vi "Create.vi"(8 "error in (no error)":errorcluster, 10 "Number of Executors":i32) -> (0 "error out":errorcluster, 3 "Executor":refnum<class "Executor.lvclass">)   [LabVIEW 2014, in "Executor.lvclass"]
uses:
  Executor.lvclass
  Controls/Executor Status - STYP.ctl
  Controls/Executor Data - STYP.ctl
  Controls/Job Results - STYP.ctl
  <vilib>/ActorFramework/Message Enqueuer/Message Enqueuer.lvclass
  Executor.lvclass/Executor.ctl
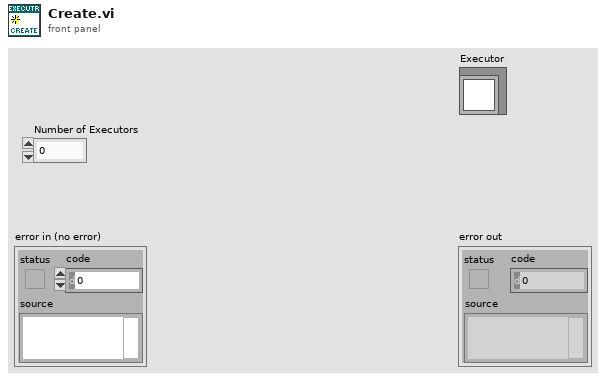
[diagram p1: front panel]
types:
  T1 = typedef "Executor Data - STYP.ctl" = cluster{"Status":T2, "Result Queue":refnum<queue>, "Actor Enquerer":refnum<class "Message Enqueuer.lvclass">}
  T2 = typedef "Executor Status - STYP.ctl" = cluster{"Executor Name":string, "Status":bool}
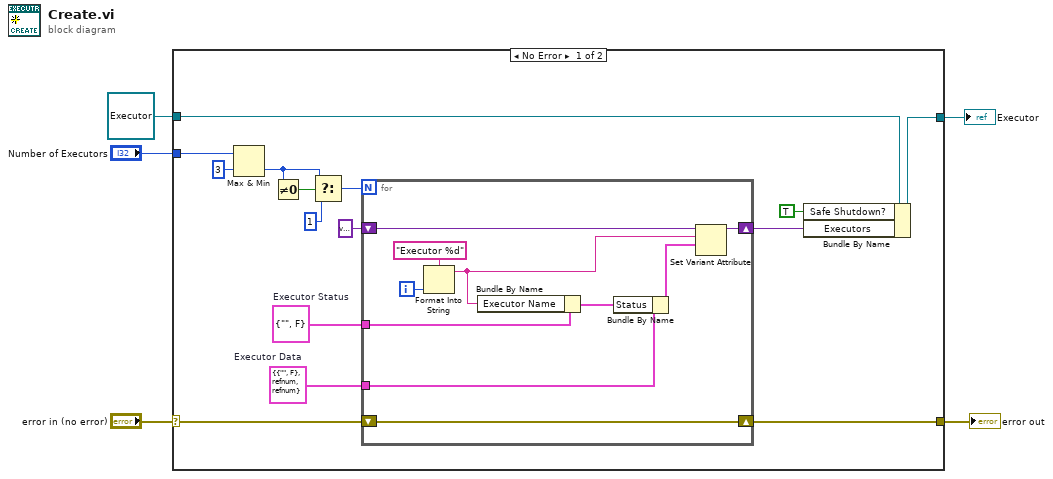
[diagram p0: block diagram]
diagram:
  n1 = case shown="No Error" "error in (no error)" {
    selector: "error in (no error)" -> [w11 w31]
    tunnel: [w10 w31] -> w4
    tunnel: [w8 _] -> w3
    tunnel: "Number of Executors" -> [w12 _]
    tunnel: refnum<class "Executor.lvclass"> refnum ("Executor.lvclass") -> [w7 _]
    frame No Error {
      w6 = T1 {"Status"={"Executor Name"="", "Status"=FALSE}, "Result Queue"=refnum, "Actor Enquerer"=refnum}  # Executor Data
      w20 = T2 {"Executor Name"="", "Status"=FALSE}  # Executor Status
      n2 = Max & Min(x=w12, y=3) -> (min(x,y)=w16:i32)  [unwired: 1 out]
      n3 = Not Equal To 0?(x=w16) -> (x != 0?=w18:bool)
      n4 = Select(t=w16, s=w18, f=1) -> (s? t:f=w15:i32)
      n5 = for {
        N: w15 -> [_]
        tunnel: w20 -> [w30]
        shift-right: [w27] -> w13
        shift-left: variant -> [w26]
        shift-right: [w23] -> w10
        shift-left: w11 -> [w23]
        tunnel: w6 -> [w21]
        i -> [w22]
        n6 = Format Into String(format string="Executor %d", w22) -> (resulting string=w28:string)  [unwired: 2 in, 1 out]
        n7 = Bundle By Name(cluster=w30, "Executor Name"=w28) -> (w24:T2)
        n8 = Bundle By Name(cluster=w21, "Status"=w24) -> (w25:T1)
        n9 = Set Variant Attribute(Variant=w26, name=w28, value=w25) -> (Variant out=w27:variant)  [unwired: 1 in, 2 out]
      }
      n10 = Bundle By Name(cluster=w7, "Safe Shutdown?"=TRUE, "Executors"=w13) -> (w8:refnum<class "Executor.lvclass">)
    }
    frame Error {
    }
  }
  "error out" <- w4
  "Executor" <- w3
